vi "Cp-Cpk Popup.vi"(8 "error in":errorcluster, 9 "ButtonPress_UI":refnum<user-event>, 10 "Measurement Names":string[](array[string]), 11 "Cp-Cpk Popup input":string[][](array[string])) -> (0 "error out":errorcluster, 3 "Cp Cpk Popup VI reference":refnum<vi>)   [LabVIEW 2019, in "ZenGage v3.0 UI.lvclass"]
uses:
  ZenGage v3.0 UI.lvclass
  <vilib>/Utility/miscctls.llb/LVRowAndColumnTypeDef.ctl
panel:
  in  "Exit":bool
  out "Popup Title":string="     USER AUTHENTICATION"
  out "Cp-Cpk Table":string[][](table)=[["0.98", "0.98", "0.91", "1.41", "0.00", "0.03", "0.03"], ["0.14", "0.14", "0.32", "0.01", "0.00", "0.05", "0.12"], ["0.02", "0.02", "0.10", "0.00", "0.00", "0.00", "0.02"], ["1.19", "3.57", "1.56", "34.24", "1152921504606846980.00", "9.47", "4.07"], ["-0.02", "1.17", "0.47", "16.07", "768614336404564.87", "0.10", "0.04"]]
  # "Measurements"
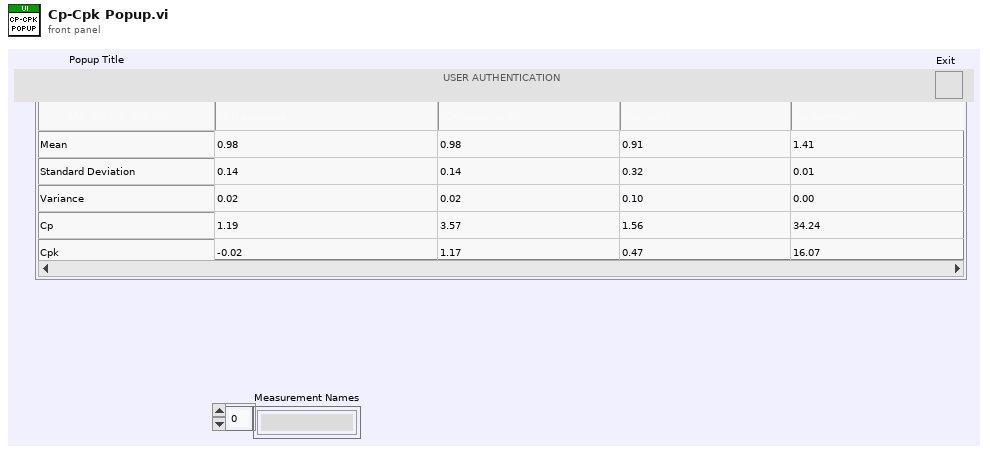
[diagram p1: front panel]
types:
  T1 = enum32{"Invalid", "Standard", "Closed", "Hidden", "Minimized", "Maximized"}
  T2 = typedef "LVRowAndColumnTypeDef.ctl" = cluster{"Row":i32, "Column":i32}
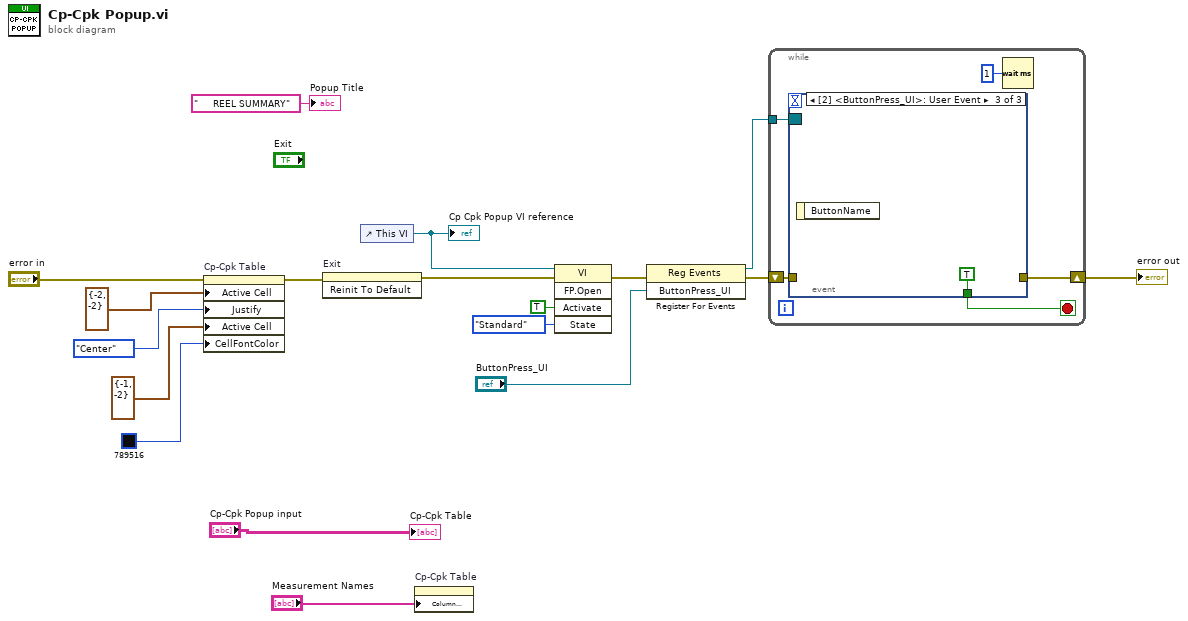
[diagram p0: block diagram]
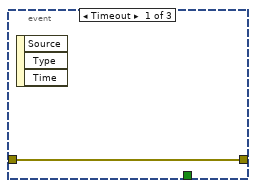
[diagram p2: hidden frame]
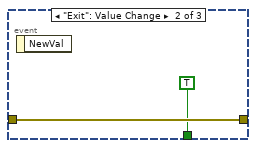
[diagram p3: hidden frame]
diagram:
  n1 = property on="Cp-Cpk Table" class="Tbl (strict)"(error in="error in", "Active Cell"=T2 {"Row"=-2, "Column"=-2} ("Active Cell:Active Cell"), "Justify"=enum16{"Left", "Center", "Right"}."Center" ("Active Cell:Cell Justification"), "Active Cell"=T2 {"Row"=-1, "Column"=-2} ("Active Cell:Active Cell"), "CellFontColor"=u32 789516) -> (error out=w10:errorcluster)  [unwired: 1 in, 1 out]
  n2 = invoke on="Exit" class="Bool" method="Reinit To Default"(error in=w10) -> (error out=w9:errorcluster)  [unwired: 2 in, 2 out]
  n3 = control-ref of="This VI"() -> (w8:refnum<vi>)
  "Cp Cpk Popup VI reference" <- w8
  n4 = property on="Cp-Cpk Table" class="Tbl (strict)"("Column Headers[]"="Measurement Names") -> ()  [unwired: 2 in, 2 out]
  n5 = invoke class="VI" method="FP.Open"(reference=w8, error in=w9, "Activate"=TRUE ("Activate?"), "State"=T1."Standard") -> (error out=w4:errorcluster)  [unwired: 1 in, 4 out]
  n6 = register-events(error in=w4, "ButtonPress_UI") -> (reference out=w1:refnum<event-registration>, error out=w3:errorcluster)  [unwired: 1 in]
  n7 = while {
    tunnel: w1 -> [w21]
    shift-right: [w23] -> w5
    shift-left: w3 -> [w22]
    stop <- w20 stop-if-true
    n8 = event shown="[2] <ButtonPress_UI>: User Event" {
      selector: w21 -> [_ _ _]
      dyn-events: _ -> [_ _ _]
      timeout: _ -> [_ _ _]
      tunnel: w22 -> [w24 w26 _]
      tunnel: [w24 w26 _] -> w23
      tunnel: [_ TRUE TRUE] -> w20
      event Timeout {
        n9 = event-data() -> ()  [unwired: 1 in, 3 out]
      }
      event "Exit": Value Change {
        n10 = event-data() -> ()  [unwired: 1 in, 1 out]
      }
      event User Event {
        n11 = event-data() -> ()  [unwired: 1 in, 1 out]
      }
    }
    n12 = Wait (ms)(milliseconds to wait=u32 1) -> ()  [unwired: 1 out]
  }
  "error out" <- w5
  "Cp-Cpk Table" <- "Cp-Cpk Popup input"
  "Popup Title" <- "     REEL SUMMARY" ("Dialog Box out")
